vi "Integration Query.vi"(8 "error in (no error)":errorcluster, 9 "Wiring":u16(ring), 10 "Element":u8=1 min=1 max=6 step=1, 11 "Universal Power Meter in":refnum<class "Universal Power Meter.lvclass">) -> (0 "error out":errorcluster, 1 "Integration State":T1, 3 "Universal Power Meter out":refnum<class "Universal Power Meter.lvclass">)   [LabVIEW 2014, in "Universal Power Meter.lvlib" / "Universal Power Meter.lvclass"]
uses:
  Universal Power Meter.lvclass
  Integration State.ctl
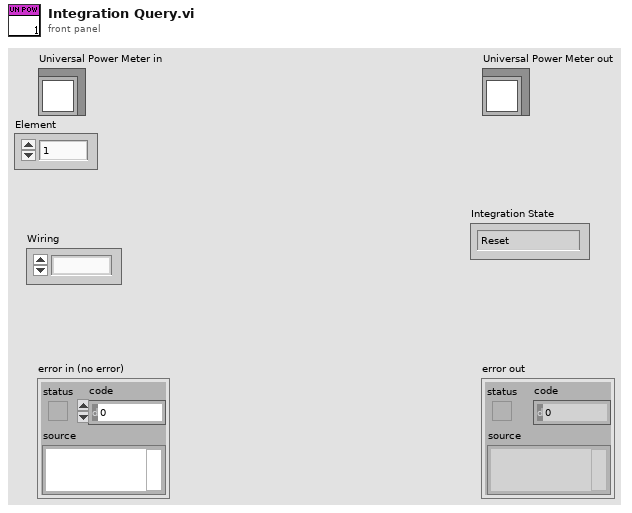
[diagram p1: front panel]
types:
  T1 = typedef "Integration State.ctl" = enum16{"Reset", "Stop", "Start"}
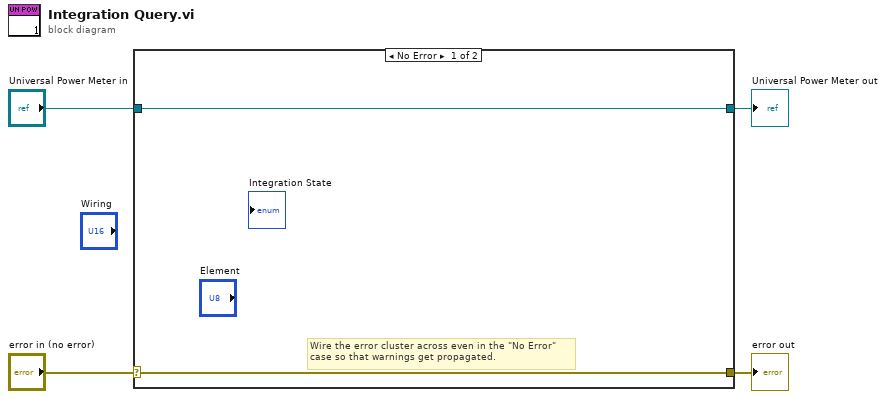
[diagram p0: block diagram]
diagram:
  n1 = case shown="No Error" "error in (no error)" {
    selector: "error in (no error)" -> [w5 w8]
    tunnel: [w5 w8] -> w3
    tunnel: [w6 w7] -> w1
    tunnel: "Universal Power Meter in" -> [w6 w7]
    frame No Error {
      # "Wire the error cluster across even in the \"No Error\"\ncase so that warnings get propagated."
    }
    frame Error {
    }
  }
  "error out" <- w3
  "Universal Power Meter out" <- w1
